vi "Trapezoidal Rule.vi"(9 "Delta_x":dbl format="%.6g", 10 "y array":dbl[](array[numeric])) -> (2 "Value of Integral":dbl format="%.10g")   [LabVIEW 2017]
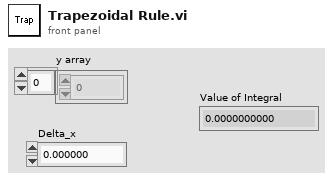
[diagram p1: front panel]
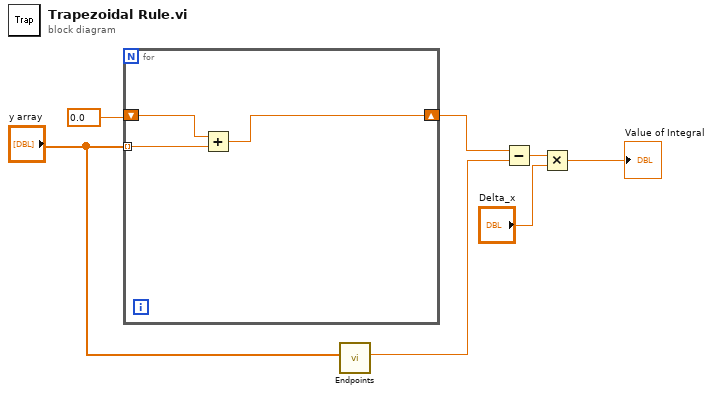
[diagram p0: block diagram]
diagram:
  n1 = for {
    shift-right: [w9] -> w2
    shift-left: 0.0 -> [w8]
    tunnel: "y array" -> [w10] mode=indexing
    n2 = Add(x=w8, y=w10) -> (x+y=w9:dbl)
  }
  n3 = call "Endpoints.vi"("Array"="y array") -> ("One-Half Engpoints Sum"=w3:dbl)  [unwired: 10 in]
  n4 = Subtract(x=w2, y=w3) -> (x-y=w1:dbl)
  n5 = Multiply(x=w1, y="Delta_x") -> (x*y=→"Value of Integral":dbl)
